vi "Agilent 3446X Series Acquire Multiple.vi"(5 "Setup":enum16{"Config+Meas", "Measure"}(ring)=enum."Measure", 6 "NPLC(10PLC)":i32=10, 7 "Sample Count (1)":i32=1, 8 "error in (no error)":errorcluster, 10 "Measurement Function (10: Voltage DC)":i32(ring)=10 items=["Continuity", "Current AC", "Current DC", "Diode", "Frequency", "Resistance 4-wire", "Period", "Resistance 2-wire", "Temperature", "Voltage AC", "Voltage DC", "Voltage DC Ratio"], 11 "VISA resource name":refnum<visa-resource-name>) -> (0 "error out":errorcluster, 2 "Measurements":dbl[](array[numeric]), 3 "mean":dbl format="%0.10f")   [LabVIEW 2019]
doc: "This example shows how to configure a measurement and take multiple readings."
uses:
  <vilib>/Analysis/baseanly.llb/Mean (DBL).vi
  <userlib>/_TI-LA/Instr Drivers/Multimeter/Agilent 3446X Series/Public/Data/Read (Multiple Points).vi
  <userlib>/_TI-LA/Instr Drivers/Multimeter/Agilent 3446X Series/Agilent 3446X Series.lvlib
  <vilib>/Analysis/NI_AALBase.lvlib
  <userlib>/_TI-LA/Instr Drivers/Multimeter/34401A/Driver/34401A.lvlib
panel:
  in  "Timeout (10000 ms)":i32=10000 format="%#.6g"
  # "(c) 2013-2015 National Instruments.  ALL RIGHTS RESERVED."
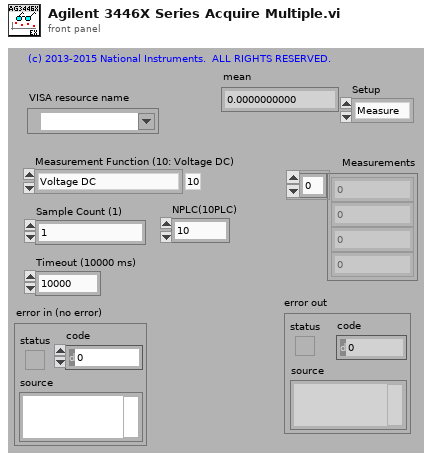
[diagram p1: front panel]
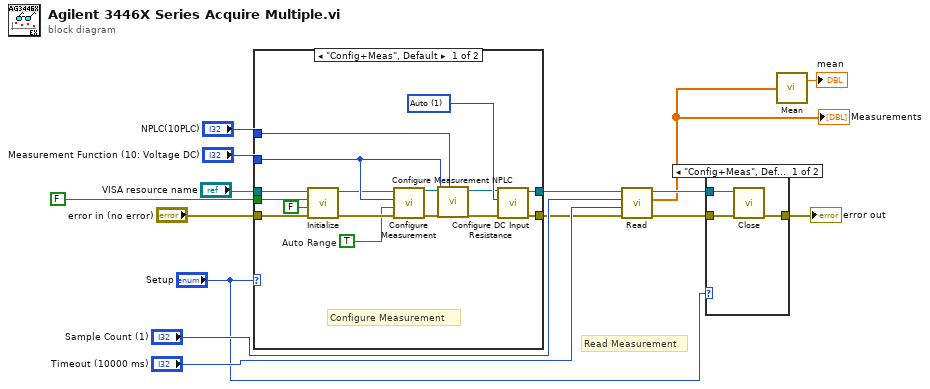
[diagram p0: block diagram]
diagram:
  # "Read Measurement"
  n1 = case shown="\"Config+Meas\", Default" "Setup" {
    tunnel: "VISA resource name" -> [w31 w33]
    tunnel: "error in (no error)" -> [w30 w32]
    tunnel: FALSE ("ID Query (True)") -> [w29 _]
    tunnel: "Measurement Function (10: Voltage DC)" -> [w28 _]
    tunnel: "NPLC(10PLC)" -> [w27 _]
    tunnel: [w26 w33] -> w3
    tunnel: [w24 w32] -> w2
    frame "Config+Meas", Default {
      w21 = TRUE  # Auto Range
      w25 = u16 1 items=["Fixed", "Auto"] ("DC Input Resistance Mode (0: Fixed)")
      # "Configure Measurement"
      n2 = call <userlib>:"Initialize.vi"("error in (no error)"=w30, "Reset (True)"=FALSE, "ID Query (True)"=w29, "VISA resource name"=w31) -> ("error out"=w22:errorcluster, "VISA resource name out"=w23:refnum<visa-resource-name>)  [unwired: 1 in, 5 out]
      n3 = call <userlib>:"Configure Measurement.vi"("error in (no error)"=w22, "Auto Range (T: Enable)"=w21, "Measurement Function (10: Voltage DC)"=w28, "VISA resource name"=w23) -> ("error out"=w19:errorcluster, "VISA resource name out"=w18:refnum<visa-resource-name>)  [unwired: 2 in, 4 out]
      n4 = call <userlib>:"Configure Measurement NPLC.vi"("NPLC(10PLC)"=w27, "error in (no error)"=w19, "Measurement Function (0: Continuity)"=w28, "VISA resource name"=w18) -> ("error out"=w16:errorcluster, "VISA resource name out"=w17:refnum<visa-resource-name>)  [unwired: 6 in]
      n5 = call <userlib>:"Configure DC Input Resistance.vi"("error in (no error)"=w16, "DC Input Resistance Mode (0: Fixed)"=w25, "VISA resource name"=w17) -> ("error out"=w24:errorcluster, "VISA resource name out"=w26:refnum<visa-resource-name>)  [unwired: 7 in]
    }
    frame "Measure" {
    }
  }
  n6 = call-poly <userlib>:"Read.vi"("error in (no error)"=w2, "Timeout (10000 ms)"="Timeout (10000 ms)", "Sample Count (1)"="Sample Count (1)", "VISA resource name"=w3) -> ("error out"=w15:errorcluster, "Measurements"=w5:dbl[], "VISA resource name out"=w14:refnum<visa-resource-name>)  [unwired: 5 out]
  "Measurements" <- w5
  n7 = case shown="\"Config+Meas\", Default" "Setup" {
    tunnel: w15 -> [w36 w37]
    tunnel: w14 -> [w35 _]
    tunnel: [w34 w37] -> w8
    frame "Config+Meas", Default {
      n8 = call <userlib>:"Close.vi"("error in (no error)"=w36, "VISA resource name"=w35) -> ("error out"=w34:errorcluster)  [unwired: 9 out]
    }
    frame "Measure" {
    }
  }
  "error out" <- w8
  n9 = call-poly <vilib>:"Mean.vi"("X"=w5) -> ("mean"=→"mean":dbl)  [unwired: 1 out]
